vi "Write Tag.vi"(8 "error in (no error)":errorcluster, 10 "Tag":string, 11 "Tree Data in":refnum<class "Tree Data.lvclass">) -> (0 "error out":errorcluster, 3 "Tree Data out":refnum<class "Tree Data.lvclass">)   [LabVIEW 2024, in "Tree Data.lvclass"]
uses:
  Tree Data.lvclass
  Tree Data.lvclass/Tree Data.ctl
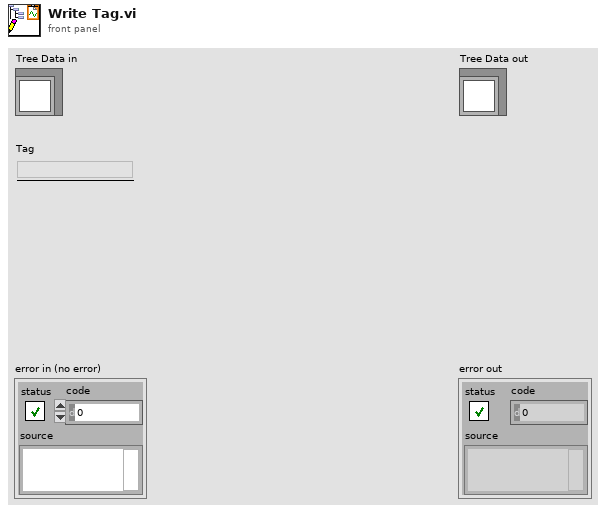
[diagram p1: front panel]
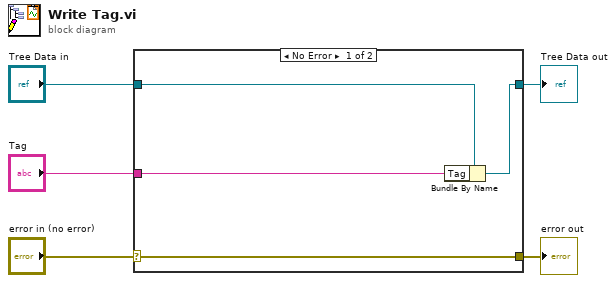
[diagram p0: block diagram]
diagram:
  n1 = case shown="No Error" "error in (no error)" {
    selector: "error in (no error)" -> [w9 w10]
    tunnel: [w9 w10] -> w4
    tunnel: [w7 w11] -> w2
    tunnel: "Tree Data in" -> [w8 w11]
    tunnel: "Tag" -> [w6 _]
    frame No Error {
      n2 = Bundle By Name(cluster=w8, "Tag"=w6) -> (w7:refnum<class "Tree Data.lvclass">)
    }
    frame Error {
    }
  }
  "error out" <- w4
  "Tree Data out" <- w2
